vi "Lvi Resistance Channel Settings.vi"(7 "NumWireType":u32, 8 "error in (no error)":errorcluster, 9 "MeasurementCurrent":dbl, 10 "Channel":u32, 11 "TaskRef":i32) -> (0 "error out":errorcluster, 2 "function return":u32(ring), 3 "TaskRef out":i32)   [LabVIEW 2022 SP3, in "DtLvLink.lvlib"]
doc: "Calls directly into the entry points of the DLL of the Data Acq SDK to set the options for resistance measurements."
uses:
  DtLvLink.lvlib
  <userlib>/LV-Link3/DtLvLink_64.dll
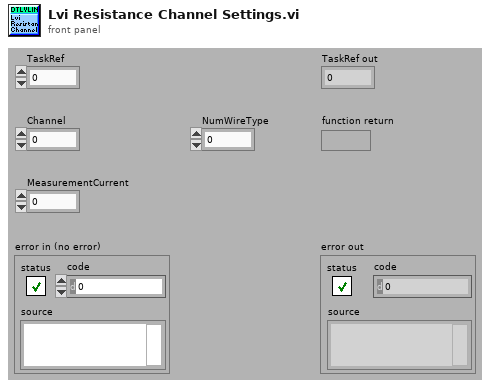
[diagram p1: front panel]
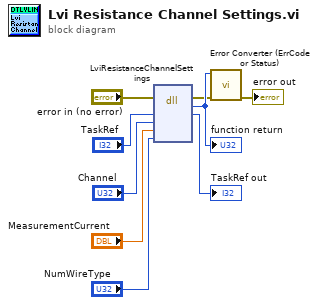
[diagram p0: block diagram]
diagram:
  n1 = dll-call lib="C:/Program Files/National Instruments/LabVIEW 2022/user.lib/LV-Link3/DtLvLink_64.*" fn="LviResistanceChannelSettings"(error in="error in (no error)", "TaskRef"="TaskRef", "Channel"="Channel", "MeasurementCurrent"="MeasurementCurrent", "NumWireType"="NumWireType") -> (error out=w2:errorcluster, w9:u32, "TaskRef"=→"TaskRef out":i32)  [unwired: 5 in, 1 out]
  "function return" <- w9
  n2 = call "Error Converter (ErrCode or Status).vi"("error in (no error)"=w2, "error code"=w9) -> ("error out"=→"error out":errorcluster)  [unwired: 9 in]
